vi "Dual Channel Temperature Log with Headers.vi"() -> ()   [LabVIEW 2014]
doc: "本VI每间隔1秒采集温度值，并持续计算最近5次温度值的平均值。本VI显示并计算原始数据和实时平均值。"
panel:
  in  "停止按钮":bool
  out "温度历史":cluster{dbl, "Temperature Value":dbl}(graph)
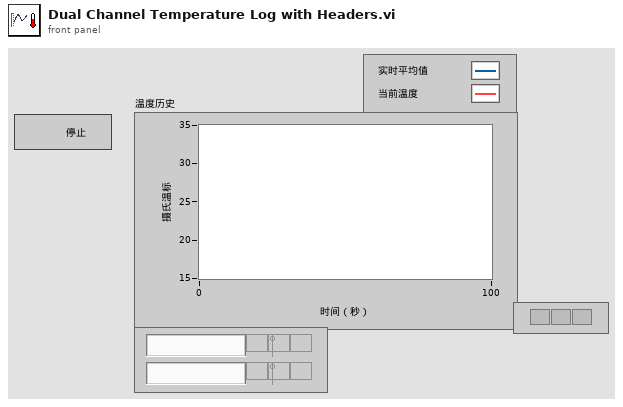
[diagram p1: front panel]
types:
  T1 = enum16{"open", "replace", "create", "open or create", "replace or create", "replace or create with confirmation"}
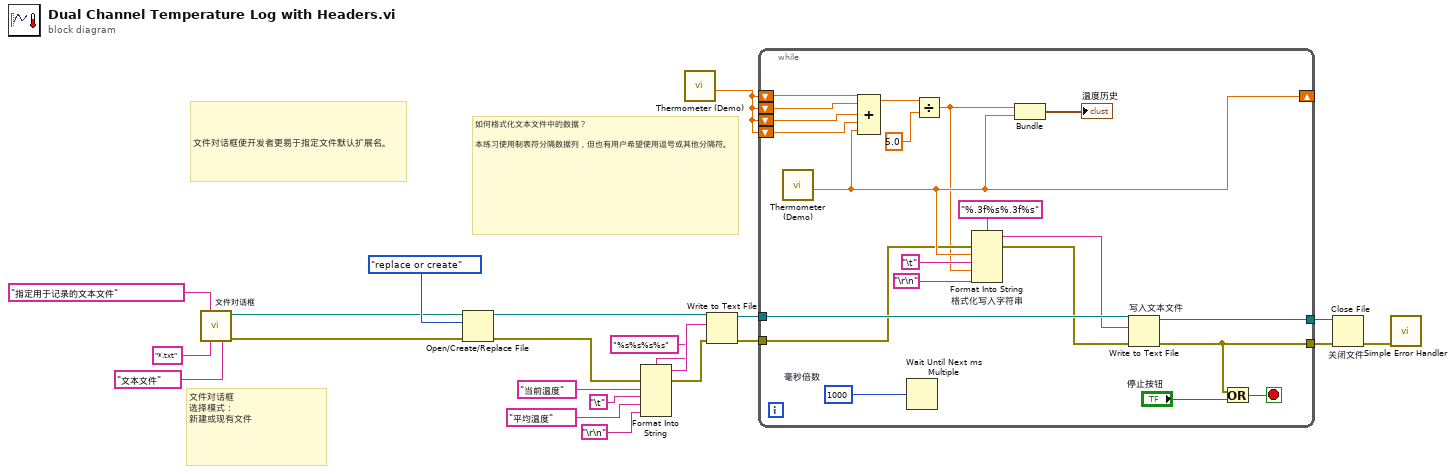
[diagram p0: block diagram]
diagram:
  # "如何格式化文本文件中的数据？\n\n本练习使用制表符分隔数据列，但也有用户希望使用逗号或其他分隔符。"
  # "文件对话框\n选择模式：\n新建或现有文件"
  # "文件对话框使开发者更易于指定文件默认扩展名。"
  n1 = call "文件对话框"("prompt"="指定用于记录的文本文件" ("类型标签"), "pattern (all files)"="*.txt" ("类型（所有文件）"), "pattern label"="文本文件" ("类型标签")) -> ("selected path"=w15:path, "error out"=w2:errorcluster)  [unwired: 9 in, 2 out]
  n2 = Open/Create/Replace File(file path (use dialog)=w15, error in=w2, operation (0:open)=T1."replace or create" ("操作(0:open)")) -> (refnum out=w16:refnum<file>, error out=w4:errorcluster)  [unwired: 4 out]
  n3 = Format Into String(format string="%s%s%s%s" ("格式字符串"), error in=w4, "当前温度" ("字符串"), "\t" ("制表符常量"), "平均温度" ("字符串"), "\r\n" ("行结束常量")) -> (resulting string=w5:string, error out=w3:errorcluster)  [unwired: 1 in]
  n4 = call "Thermometer (Demo).vi"() -> ("温度值"=w21:dbl)  [unwired: 11 in]
  n5 = Write to Text File(file (use dialog)=w16, text=w5, error in=w3) -> (refnum out=w12:refnum<file>, error out=w11:errorcluster)  [unwired: 2 out]
  n6 = while {
    shift-right: [w29] -> _
    shift-left: w21 -> [w41]
    shift-left: w21 -> [w40]
    shift-left: w21 -> [w37]
    shift-left: w21 -> [w36]
    tunnel: w11 -> [w27]
    tunnel: [w32] -> w19
    tunnel: w12 -> [w34]
    tunnel: [w33] -> w18
    stop <- w30 stop-if-true
    w42 = u32 1000  # 毫秒倍数
    n7 = call "Thermometer (Demo).vi"() -> ("温度值"=w29:dbl)  [unwired: 11 in]
    n8 = Compound Arithmetic op=ADD(w41, w40, w37, w36, w29) -> (w39:dbl)
    n9 = Wait Until Next ms Multiple(millisecond multiple=w42) -> ()  [unwired: 1 out]
    n10 = Divide(x=w39, y=5.0) -> (x/y=w23:dbl)
    n11 = Format Into String "格式化写入字符串"(format string="%.3f%s%.3f%s" ("格式字符串"), error in=w27, w29, "\t" ("制表符常量"), w23, "\r\n" ("行结束常量")) -> (resulting string=w28:string, error out=w26:errorcluster)  [unwired: 1 in]
    n12 = Bundle(w23, "温度值"=w29) -> (→"温度历史":cluster{dbl, "温度值":dbl})  [unwired: 1 in]
    n13 = Write to Text File "写入文本文件"(file (use dialog)=w34, text=w28, error in=w26) -> (refnum out=w33:refnum<file>, error out=w32:errorcluster)  [unwired: 2 out]
    n14 = Or(x=w32, y="停止按钮") -> (x .or. y?=w30:bool)
  }
  n15 = Close File "关闭文件"(refnum=w18, error in=w19) -> (error out=w20:errorcluster)  [unwired: 1 out]
  n16 = call <vilib>:"Simple Error Handler.vi"("error in (no error)"=w20) -> ()  [unwired: 1 in, 8 out]
